vi "Problem 3.vi"() -> ()   [LabVIEW 2025]
uses:
  <vilib>/gmath/NI_AAL_MathFunc.lvlib
panel:
  in  "n":i64=600851475143
  out "Largest Prime Factor":i64
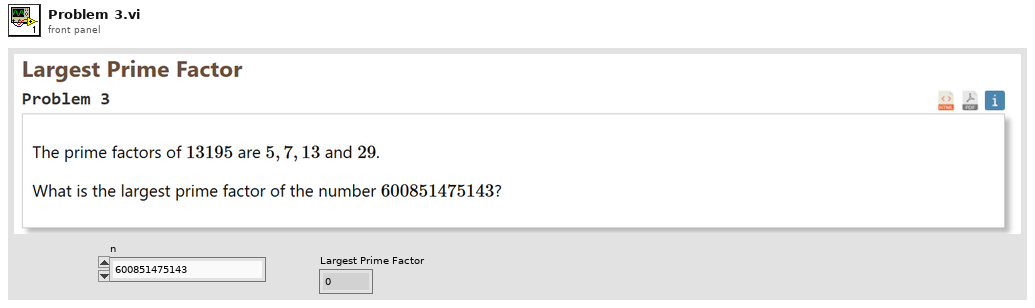
[diagram p1: front panel]
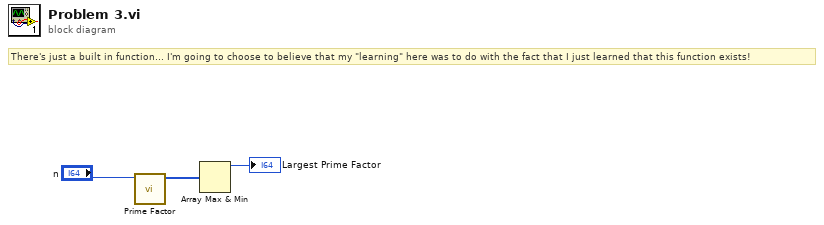
[diagram p0: block diagram]
diagram:
  # "There's just a built in function... I'm going to choose to believe that my \"learning\" here was to do with the fact that I just learned that this function exists!"
  n1 = call <vilib>:"Prime Factor.vi"("n"="n") -> ("Prime Factors"=w2:i64[])  [unwired: 9 in]
  n2 = Array Max & Min(array=w2) -> (max value=→"Largest Prime Factor":i64)  [unwired: 3 out]
